vi "Write Number of Tatics.vi"(8 "error in (no error)":errorcluster, 10 "Number of Tatics":dbl=1.0, 11 "WaitPassRole in":refnum<class "WaitPassRole.lvclass">) -> (0 "error out":errorcluster, 3 "WaitPassRole out":refnum<class "WaitPassRole.lvclass">)   [LabVIEW 2024, in "WaitPassRole.lvclass"]
uses:
  WaitPassRole.lvclass
  WaitPassRole.lvclass/WaitPassRole.ctl
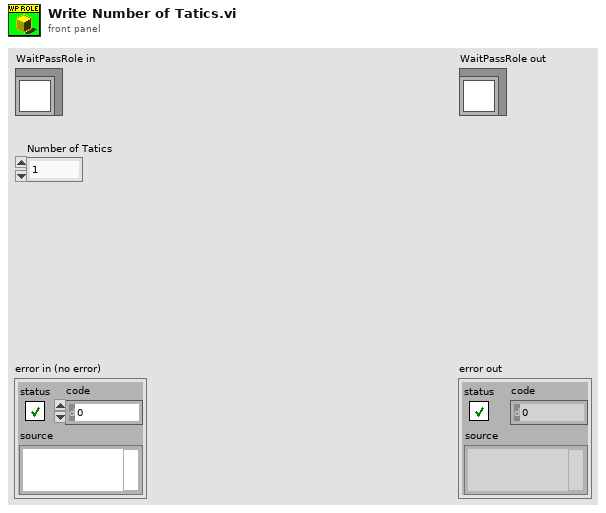
[diagram p1: front panel]
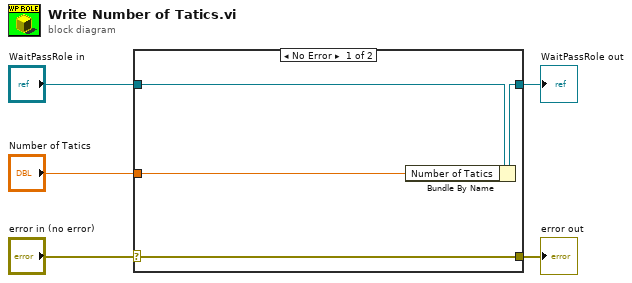
[diagram p0: block diagram]
diagram:
  n1 = case shown="No Error" "error in (no error)" {
    selector: "error in (no error)" -> [w9 w10]
    tunnel: [w9 w10] -> w4
    tunnel: [w7 w11] -> w2
    tunnel: "WaitPassRole in" -> [w8 w11]
    tunnel: "Number of Tatics" -> [w6 _]
    frame No Error {
      n2 = Bundle By Name(cluster=w8, "Number of Tatics"=w6) -> (w7:refnum<class "WaitPassRole.lvclass">)
    }
    frame Error {
    }
  }
  "error out" <- w4
  "WaitPassRole out" <- w2
